vi "newWorkingPair.vi"(8 "Error (Input)":errorcluster, 11 "WorkingPair (Input)":T1={"no_iso"=1, "no_p_sat"=1, "path_db"="D:\\Driesel\\SorpLibLocal\\LabVIEW_wrapper\\data\\json\\sorpproplib_minimalExample.json", "wp_as"="silicagel", "wp_st"="123", "wp_iso"="DubininArctan1", "wp_rf"="water", "rf_rhol"="SaturatedLiquidDensity_EoS1", "no_rhol"=1, "rf_psat"="VaporPressure_EoS1"}) -> (0 "Error (Output)":errorcluster caption="Error(Output)", 3 "workingPair":i64)   [LabVIEW 2017]
doc: "newWorkingPair:\n * ---------------\n *\n * Initialization function to create a new WorkingPair-struct. Therefore,\n * function checks first if enough memory available to allocate WorkingPair-\n * struct and then reads coefficients of functions from database and sets\n * pointers within the struct depending on working pair given as input.\n * If memory allocation fails, functions returns NULL and prints a warning.\n *\n * Parameters:\n * -----------\n * const char *path_db:\n * Path to database.\n * const char *wp_as:\n * Name of sorbent.\n * const char *wp_st:\n * Name of sub-type of sorbent.\n * const char *wp_rf:\n * Name of refrigerant.\n * const char *wp_iso:\n * Name of isotherm.\n * int no_iso:\n * ID of isotherm (i.e. when more than one isotherm is available)\n * const char *rf_psat:\n * Name of calculation approach for vapor pressure.\n * int no_p_sat:\n * ID of vapor pressure equation (i.e. when more than one equation is\n * available)\n * const char *rf_rhol:\n * Name of calculation approach for liquid density.\n * int no_rhol:\n * ID of liquid density equation (i.e. when more than one equation is\n * available)\n *\n * Returns:\n * --------\n * struct *WorkingPair:\n * Returns malloc-ed WorkingPair-struct containing all information required\n * to calculate the resorption equilibrium of the working working.\n *\n * History:\n * --------\n * 07/13/2021, by Jannik Driesel (supervised by Mirko Engelpracht):\n * First implementation."
uses:
  data/win32bit/libsorpPropLib.dll
panel:
  # "Path to database"
  # "Name of sorbent"
  # "Name of sub-type of sorbent"
  # "Name of refrigerant"
  # "Name of isotherm"
  # "ID of isotherm"
  # "Name of calculation approach for vapor pressure"
  # "ID of vapor pressure equation"
  # "Name of calculation approach for liquid density"
  # "ID of liquid density equation"
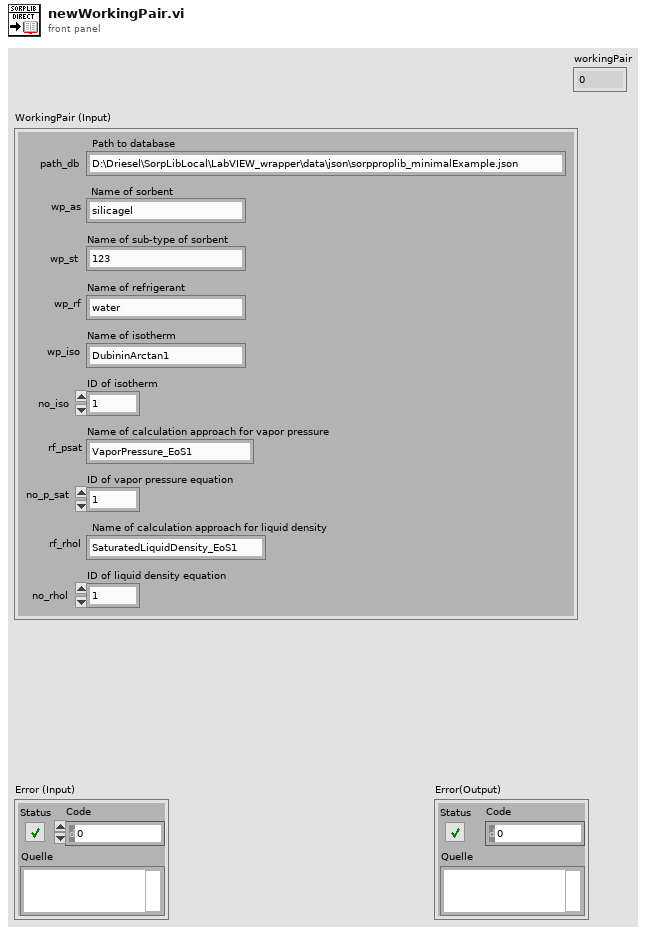
[diagram p1: front panel]
types:
  T1 = cluster{"no_iso":i32, "no_p_sat":i32, "path_db":string, "wp_as":string, "wp_st":string, "wp_iso":string, "wp_rf":string, "rf_rhol":string, "no_rhol":i32, "rf_psat":string}
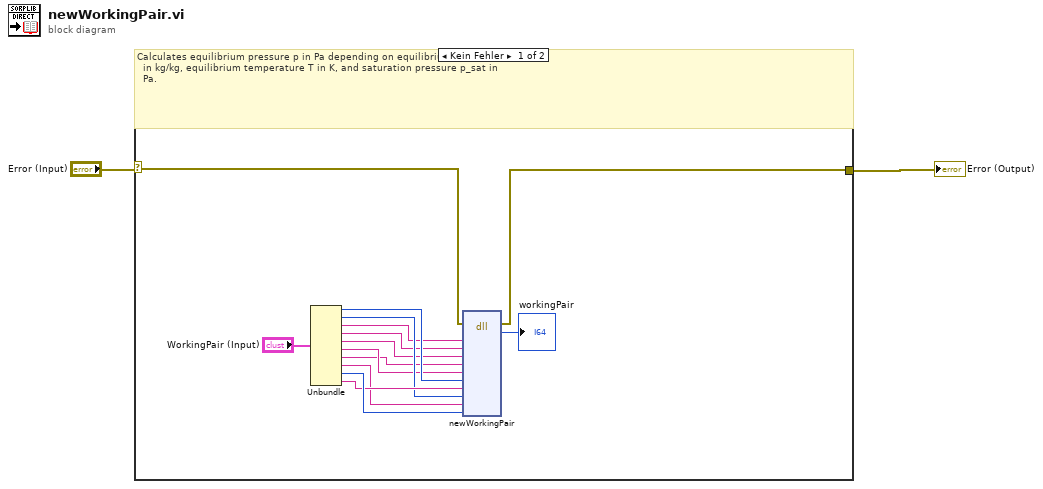
[diagram p0: block diagram]
diagram:
  n1 = case shown="Kein Fehler" "Error (Input)" {
    selector: "Error (Input)" -> [w5 w17]
    tunnel: [w4 w17] -> w1
    frame No Error {
      # "Calculates equilibrium pressure p in Pa depending on equilibrium loading w\n  in kg/kg, equilibrium temperature T in K, and saturation pressure p_sat in\n  Pa."
      n2 = Unbundle("WorkingPair (Input)") -> ("no_iso"=w13:i32, "no_p_sat"=w14:i32, "path_db"=w7:string, "wp_as"=w8:string, "wp_st"=w9:string, "wp_iso"=w11:string, "wp_rf"=w10:string, "rf_rhol"=w12:string, "no_rhol"=w16:i32, "rf_psat"=w15:string)
      n3 = dll-call lib="D:/Driesel/SorpLibLocal/LabVIEW_wrapper/data/win32bit/libsorpPropLib.dll" fn="newWorkingPair"(error in=w5, "path_db"=w7, "wp_as"=w8, "wp_st"=w9, "wp_rf"=w10, "wp_iso"=w11, "no_iso"=w13, "rf_psat"=w15, "no_p_sat"=w14, "rf_rhol"=w12, "no_rhol"=w16) -> (error out=w4:errorcluster, "workingPair"=→"workingPair":i64)  [unwired: 12 in, 1 out]
    }
    frame Error {
      # "Error - No calculations"
    }
  }
  "Error (Output)" <- w1
